vi "test_AK RS-xxx Read.vi"(8 "error in (no error)":errorcluster, 11 "TestCase in":refnum<class "Instrument Addon Serial Protocols Unit Tests.lvclass">) -> (0 "error out":errorcluster, 3 "TestCase out":refnum<class "Instrument Addon Serial Protocols Unit Tests.lvclass">)   [LabVIEW 2023, in "Instrument Addon Serial Protocols Unit Tests.lvclass"]
uses:
  Instrument Addon Serial Protocols Unit Tests.lvclass
  Instrument Addon Serial Protocols Unit Tests.lvclass/Instrument Addon Serial Protocols Unit Tests.ctl
  <vilib>/addons/_JKI Toolkits/VI Tester/TestCase.llb/TestCase.lvclass
  AK RS-xxx/AK RS-xxx.lvclass
  Protocol Parent/Methods/Read Parameter.ctl
  Protocol Parent/Protocol Parent.lvclass
  Listener/ListenerClassControls/Operation.ctl
  Listener/Listener.lvclass
  Constants.vi
  <vilib>/platform/TimedLoop/XDataNode/XDataNode.xnode
  <vilib>/Platform/TimedLoop/XDataNode/timing_clust.ctl
  <vilib>/Platform/TimedLoop/XDataNode/XDNodeRunTimeDep.lvlib
  <vilib>/Platform/TimedLoop/XDataNode/wakeup.ctl
  <vilib>/Platform/TimedLoop/XDataNode/nitl_modes.ctl
  RS-xxx/RS-xxx.lvclass
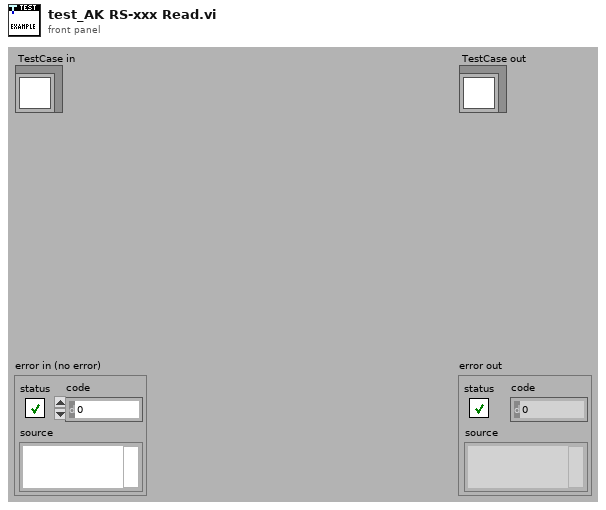
[diagram p1: front panel]
types:
  T1 = typedef "Protocols.lvlib/Protocol Parent.lvclass/Read Parameter.ctl" = cluster{"Wait Type":enum16{"Byte Count", "Wait sec"}, "Wait Value":dbl}
  T2 = typedef "Listener.lvclass/Operation.ctl" = enum16{"Read", "Write"}
  T3 = typedef "XDNodeRunTimeDep.lvlib/timing_clust.ctl" = cluster{"Expected End [f-1]":u64, "Actual End [f-1]":u64, "Finished Late? [f-1]":bool, "Expected End [i-1]":u64, "Actual End [i-1]":u64, "Finished Late? [i-1]":bool, "Expected Start [i]":u64, "Actual Start [i]":u64, "Expected Start [f]":u64, "Actual Start [f]":u64, "Source Name":string, "Structure Name":string, "Period":i64, "Deadline":i64, "Offset":i64, "Start":i64, "Priority":i32, "Timeout":i32, "Mode":T4, "Wakeup Reason":T5, "Error":errorcluster, "Source Type":string, "Secondary Source Type":string, "Global End Time":u64, "Global Start Time":u64, "Frame Duration":u64, "Iteration Duration":u64, "Assigned CPU":i32, "I/O Scan Engine Mode":u32}
  T4 = typedef "XDNodeRunTimeDep.lvlib/nitl_modes.ctl" = enum32{"No Change", "Process missed periods, maintain original phase", "Discard missed periods, maintain original phase", "Process missed periods, ignore original phase", "Discard missed periods, ignore original phase"}
  T5 = typedef "XDNodeRunTimeDep.lvlib/wakeup.ctl" = enum32{"Normal", "Aborted", "Asynchronous wakeup", "Timing source error", "Timed loop error", "Timeout"}
  T6 = typedef "Listener.lvclass/RS-xxx Data Structure.ctl" = cluster{"Virtual COM Port Settings 1":cluster{"Port":string, "Baud Rate":u32, "Data Bits":u16, "Parity":enum16{"None", "Odd", "Even", "Mark", "Space"}, "Stop Bits":u16, "Flow Control":u16, "XON":enum16{"NUL", "SOH", "STX", "ETX", "EOT", "ENQ", "ACK", "BEL", "BS", "HT", "LF", "VT", "FF", "CR", "SO", "SI", "DLE", "DC1", "DC2", "DC3", "DC4", "NAK", "SYN", "ETB", "CAN", "EM", "SUB", "ESC", "FS", "GS", "RS", "US", "SP", "!", "\"", "#", "$", "%", "&", "'", "(", ")", "*", "+", ",", "- (-)", ".", "/", "0", "1", "2", "3", "4", "5", "6", "7", "8", "9", ":", ";", "<", "=", ">", "?", "@", "A", "B", "C", "D", "E", "F", "G", "H", "I", "J", "K", "L", "M", "N", "O", "P", "Q", "R", "S", "T", "U", "V", "W", "X", "Y", "Z", "[", "\\", "]", "^", "_", "`", "a", "b", "c", "d", "e", "f", "g", "h", "i", "j", "k", "l", "m", "n", "o", "p", "q", "r", "s", "t", "u", "v", "w", "x", "y", "z", "{", "|", "}", "~"}, "XOFF":enum16{"NUL", "SOH", "STX", "ETX", "EOT", "ENQ", "ACK", "BEL", "BS", "HT", "LF", "VT", "FF", "CR", "SO", "SI", "DLE", "DC1", "DC2", "DC3", "DC4", "NAK", "SYN", "ETB", "CAN", "EM", "SUB", "ESC", "FS", "GS", "RS", "US", "SP", "!", "\"", "#", "$", "%", "&", "'", "(", ")", "*", "+", ",", "- (-)", ".", "/", "0", "1", "2", "3", "4", "5", "6", "7", "8", "9", ":", ";", "<", "=", ">", "?", "@", "A", "B", "C", "D", "E", "F", "G", "H", "I", "J", "K", "L", "M", "N", "O", "P", "Q", "R", "S", "T", "U", "V", "W", "X", "Y", "Z", "[", "\\", "]", "^", "_", "`", "a", "b", "c", "d", "e", "f", "g", "h", "i", "j", "k", "l", "m", "n", "o", "p", "q", "r", "s", "t", "u", "v", "w", "x", "y", "z", "{", "|", "}", "~"}, "End Read on Termination Character":bool, "End Write on Termination Character":bool, "Termination Character":u8}, "Virtual COM Port Settings 2":cluster{"Port":string, "Baud Rate":u32, "Data Bits":u16, "Parity":enum16{"None", "Odd", "Even", "Mark", "Space"}, "Stop Bits":u16, "Flow Control":u16, "XON":enum16{"NUL", "SOH", "STX", "ETX", "EOT", "ENQ", "ACK", "BEL", "BS", "HT", "LF", "VT", "FF", "CR", "SO", "SI", "DLE", "DC1", "DC2", "DC3", "DC4", "NAK", "SYN", "ETB", "CAN", "EM", "SUB", "ESC", "FS", "GS", "RS", "US", "SP", "!", "\"", "#", "$", "%", "&", "'", "(", ")", "*", "+", ",", "- (-)", ".", "/", "0", "1", "2", "3", "4", "5", "6", "7", "8", "9", ":", ";", "<", "=", ">", "?", "@", "A", "B", "C", "D", "E", "F", "G", "H", "I", "J", "K", "L", "M", "N", "O", "P", "Q", "R", "S", "T", "U", "V", "W", "X", "Y", "Z", "[", "\\", "]", "^", "_", "`", "a", "b", "c", "d", "e", "f", "g", "h", "i", "j", "k", "l", "m", "n", "o", "p", "q", "r", "s", "t", "u", "v", "w", "x", "y", "z", "{", "|", "}", "~"}, "XOFF":enum16{"NUL", "SOH", "STX", "ETX", "EOT", "ENQ", "ACK", "BEL", "BS", "HT", "LF", "VT", "FF", "CR", "SO", "SI", "DLE", "DC1", "DC2", "DC3", "DC4", "NAK", "SYN", "ETB", "CAN", "EM", "SUB", "ESC", "FS", "GS", "RS", "US", "SP", "!", "\"", "#", "$", "%", "&", "'", "(", ")", "*", "+", ",", "- (-)", ".", "/", "0", "1", "2", "3", "4", "5", "6", "7", "8", "9", ":", ";", "<", "=", ">", "?", "@", "A", "B", "C", "D", "E", "F", "G", "H", "I", "J", "K", "L", "M", "N", "O", "P", "Q", "R", "S", "T", "U", "V", "W", "X", "Y", "Z", "[", "\\", "]", "^", "_", "`", "a", "b", "c", "d", "e", "f", "g", "h", "i", "j", "k", "l", "m", "n", "o", "p", "q", "r", "s", "t", "u", "v", "w", "x", "y", "z", "{", "|", "}", "~"}, "End Read on Termination Character":bool, "End Write on Termination Character":bool, "Termination Character":u8}, "Data":string, "Data Length":u32}
  T7 = cluster{"Port":string, "Baud Rate":u32, "Data Bits":u16, "Parity":enum16{"None", "Odd", "Even", "Mark", "Space"}, "Stop Bits":u16, "Flow Control":u16, "XON":enum16{"NUL", "SOH", "STX", "ETX", "EOT", "ENQ", "ACK", "BEL", "BS", "HT", "LF", "VT", "FF", "CR", "SO", "SI", "DLE", "DC1", "DC2", "DC3", "DC4", "NAK", "SYN", "ETB", "CAN", "EM", "SUB", "ESC", "FS", "GS", "RS", "US", "SP", "!", "\"", "#", "$", "%", "&", "'", "(", ")", "*", "+", ",", "- (-)", ".", "/", "0", "1", "2", "3", "4", "5", "6", "7", "8", "9", ":", ";", "<", "=", ">", "?", "@", "A", "B", "C", "D", "E", "F", "G", "H", "I", "J", "K", "L", "M", "N", "O", "P", "Q", "R", "S", "T", "U", "V", "W", "X", "Y", "Z", "[", "\\", "]", "^", "_", "`", "a", "b", "c", "d", "e", "f", "g", "h", "i", "j", "k", "l", "m", "n", "o", "p", "q", "r", "s", "t", "u", "v", "w", "x", "y", "z", "{", "|", "}", "~"}, "XOFF":enum16{"NUL", "SOH", "STX", "ETX", "EOT", "ENQ", "ACK", "BEL", "BS", "HT", "LF", "VT", "FF", "CR", "SO", "SI", "DLE", "DC1", "DC2", "DC3", "DC4", "NAK", "SYN", "ETB", "CAN", "EM", "SUB", "ESC", "FS", "GS", "RS", "US", "SP", "!", "\"", "#", "$", "%", "&", "'", "(", ")", "*", "+", ",", "- (-)", ".", "/", "0", "1", "2", "3", "4", "5", "6", "7", "8", "9", ":", ";", "<", "=", ">", "?", "@", "A", "B", "C", "D", "E", "F", "G", "H", "I", "J", "K", "L", "M", "N", "O", "P", "Q", "R", "S", "T", "U", "V", "W", "X", "Y", "Z", "[", "\\", "]", "^", "_", "`", "a", "b", "c", "d", "e", "f", "g", "h", "i", "j", "k", "l", "m", "n", "o", "p", "q", "r", "s", "t", "u", "v", "w", "x", "y", "z", "{", "|", "}", "~"}, "End Read on Termination Character":bool, "End Write on Termination Character":bool, "Termination Character":u8}
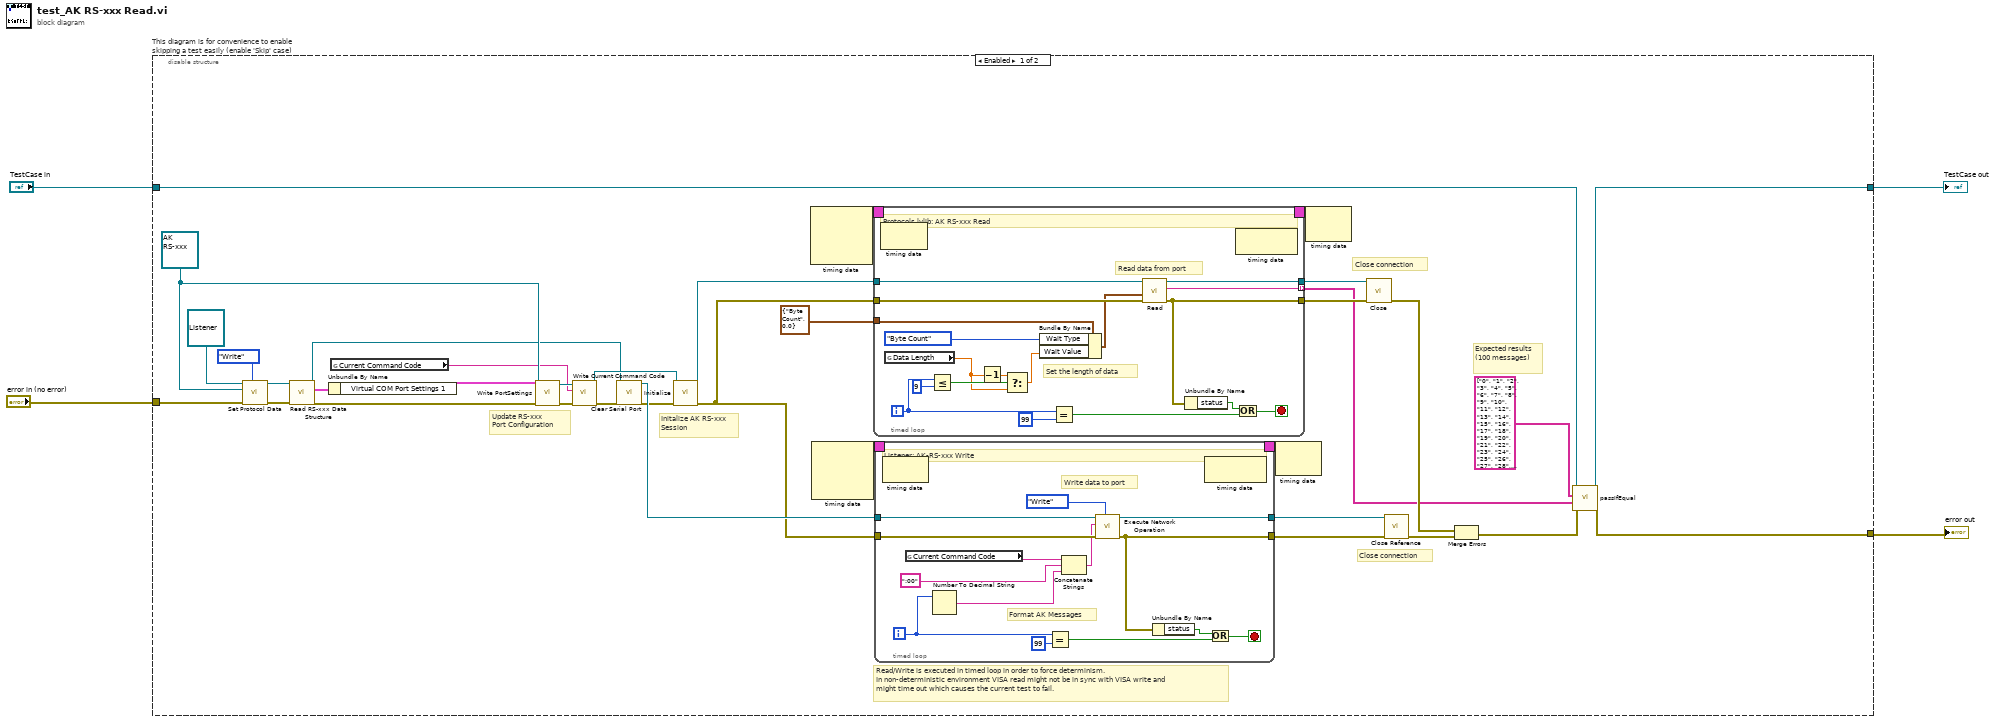
[diagram p0: block diagram]
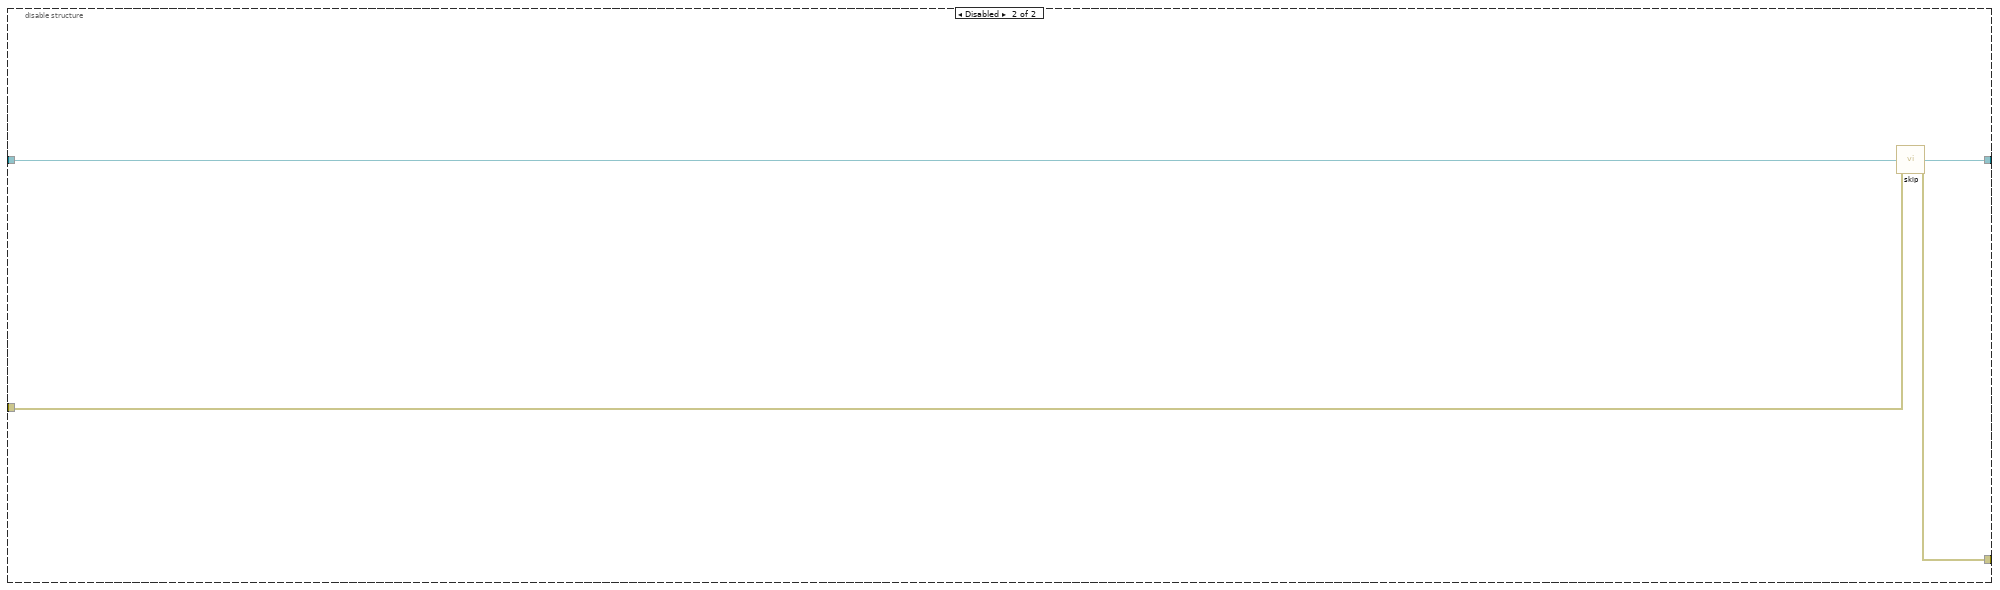
[diagram p2: hidden frame]
diagram:
  n1 = disable-structure "This diagram is for convenience to enable skipping a test easily (enable 'Skip' case)" shown="Enabled" {
    disable-tunnel: "TestCase in" -> [w40 w84]
    disable-tunnel: [w39 w82] -> w1
    disable-tunnel: [w38 w83] -> w3
    disable-tunnel: "error in (no error)" -> [w37 w81]
    frame Enabled {
      w19 = refnum<class "AK RS-xxx.lvclass"> refnum ("Protocols.lvlib:AK RS-xxx.lvclass")
      # "Update RS-xxx \nPort Configuration"
      # "Initalize AK RS-xxx\nSession"
      # "Close connection"
      # "Close connection"
      # "Expected results\n(100 messages)"
      # "Read/Write is executed in timed loop in order to force determinism.\nIn non-deterministic environment VISA read might not be in sync with VISA write and\nmight time out which causes the current test to fail."
      n2 = call "Set Protocol Data.vi"("Operation"=Operation."Write", "error in (no error)"=w37, "Protocols.lvlib:Protocol Parent.lvclass"=w19, "Listener In.lvclass"=refnum<class "Listener.lvclass"> refnum ("Listener.lvclass")) -> ("error out"=w23:errorcluster, "Listener Out.lvclass"=w24:refnum<class "Listener.lvclass">)  [unwired: 6 in]
      n3 = call-dynamic "Read RS-xxx Data Structure.vi"("error in (no error)"=w23, "Listener in"=w24) -> ("error out"=w12:errorcluster, "RS-xxx Data Structure"=w22:T6, "Listener out"=w10:refnum<class "Listener.lvclass">)  [unwired: 7 in]
      n4 = Unbundle By Name(w22) -> ("Virtual COM Port Settings 1"=w18:T7)
      n5 = global read "Constants.vi" "Current Command Code"() -> (w15:string)
      n6 = call "Write PortSettings.vi"("error in (no error)"=w12, "PortSettings"=w18, "RS232 in"=w19) -> ("error out"=w16:errorcluster, "RS232 out"=w17:refnum<class "AK RS-xxx.lvclass">)  [unwired: 7 in]
      n7 = call "Write Current Command Code.vi"("error in (no error)"=w16, "Current Command Code"=w15, "AK RS232 in"=w17) -> ("error out"=w11:errorcluster, "AK RS232 out"=w14:refnum<class "AK RS-xxx.lvclass">)  [unwired: 7 in]
      n8 = call "Clear Serial Port.vi"("error in (no error)"=w11, "Listener In.lvclass"=w10) -> ("error out"=w7:errorcluster, "Listener out"=w9:refnum<class "Listener.lvclass">)  [unwired: 8 in]
      n9 = call-dynamic "Initialize.vi"("error in (no error)"=w7, "RS232 in"=w14) -> ("error out"=w8:errorcluster, "RS232 out"=w13:refnum<class "AK RS-xxx.lvclass">)  [unwired: 8 in]
      n10 = node-c288() -> (w34:T3)  [unwired: 3 in]
      n11 = node-c288() -> (w36:T3)  [unwired: 3 in]
      n12 = timed-loop {
        timing: w34 -> [_]
        timing-out: [_] -> w33
        tunnel: T1 {"Wait Type"=enum."Byte Count", "Wait Value"=0.0} ("Read Parameter") -> [w52]
        tunnel: [w49] -> w6 mode=indexing
        tunnel: [w50] -> w20
        tunnel: w13 -> [w43]
        tunnel: w8 -> [w55]
        tunnel: [w42] -> w27
        i -> [w44]
        stop <- w56 stop-if-true
        # "Set the length of data"
        # "Read data from port"
        # "Protocols.lvlib: AK RS-xxx Read"
        n13 = node-c288() -> ()  [unwired: 1 in, 1 out]
        n14 = global read "Constants.vi" "Data Length"() -> (w48:dbl)
        n15 = Less Or Equal?(x=w44, y=9) -> (x <= y?=w53:bool)
        n16 = Decrement(x=w48) -> (x-1=w46:dbl)
        n17 = Select(t=w46, s=w53, f=w48) -> (s? t:f=w47:dbl)
        n18 = Bundle By Name(cluster=w52, "Wait Type"=enum16{"Byte Count", "Wait sec"}."Byte Count", "Wait Value"=w47) -> (w51:T1)
        n19 = Equal?(x=w44, y=99) -> (x = y?=w58:bool)
        n20 = call-dynamic "Read.vi"("error in (no error)"=w55, "Variant"=w51, "AK RS232 in"=w43) -> ("error out"=w42:errorcluster, "String"=w49:string, "AK RS232 out"=w50:refnum<class "AK RS-xxx.lvclass">)  [unwired: 6 in]
        n21 = Unbundle By Name(w42) -> ("status"=w41:bool)
        n22 = node-c288() -> ()  [unwired: 1 in, 1 out]
        n23 = Or(x=w41, y=w58) -> (x .or. y?=w56:bool)
      }
      n24 = timed-loop {
        timing: w36 -> [_]
        timing-out: [_] -> w35
        tunnel: w9 -> [w72]
        tunnel: [w73] -> w26
        tunnel: w8 -> [w71]
        tunnel: [w64] -> w25
        i -> [w67]
        stop <- w74 stop-if-true
        # "Format AK Messages"
        # "Write data to port"
        # "Listener: AK-RS-xxx Write"
        n25 = node-c288() -> ()  [unwired: 1 in, 1 out]
        n26 = global read "Constants.vi" "Current Command Code"() -> (w68:string)
        n27 = Number To Decimal String(number=w67) -> (decimal integer string=w69:string)  [unwired: 1 in]
        n28 = Equal?(x=w67, y=99) -> (x = y?=w75:bool)
        n29 = Concatenate Strings(w68, ":00", w69) -> (w66:string)
        n30 = call "Execute Network Operation.vi"("Operation"=Operation."Write", "error in (no error)"=w71, "Message"=w66, "Listener In.lvclass"=w72) -> ("error out"=w64:errorcluster, "Listener Out.lvclass"=w73:refnum<class "Listener.lvclass">)  [unwired: 6 in]
        n31 = Unbundle By Name(w64) -> ("status"=w63:bool)
        n32 = node-c288() -> ()  [unwired: 1 in, 1 out]
        n33 = Or(x=w63, y=w75) -> (x .or. y?=w74:bool)
      }
      n34 = node-c288(w35) -> ()  [unwired: 1 out]
      n35 = node-c288(w33) -> ()  [unwired: 1 out]
      n36 = call-dynamic "Close.vi"("error in (no error)"=w27, "RS232 in"=w20) -> ("error out"=w29:errorcluster)  [unwired: 8 in, 1 out]
      n37 = call "Close Reference.vi"("error in (no error)"=w25, "Listener In.lvclass"=w26) -> ("error out"=w28:errorcluster)  [unwired: 8 in, 1 out]
      n38 = Merge Errors(w29, w28) -> (w30:errorcluster)
      n39 = call-dynamic "passIfEqual.vi"("error in (no error)"=w30, "y"=w6, "x"=string[] ["0", "1", "2", "3", "4", "5", "6", "7", "8", "9", "10", "11", "12", "13", "14", "15", "16", "17", "18", "19", "20", "21", "22", "23", "24", "25", "26", "27", "28", "29", "30", "31", "32", "33", "34", "35", "36", "37", "38", "39", "40", "41", "42", "43", "44", "45", "46", "47", "48", "49", "50", "51", "52", "53", "54", "55", "56", "57", "58", "59", "60", "61", "62", "63", "64", "65", "66", "67", "68", "69", "70", "71", "72", "73", "74", "75", "76", "77", "78", "79", "80", "81", "82", "83", "84", "85", "86", "87", "88", "89", "90", "91", "92", "93", "94", "95", "96", "97", "98", "99"] ("Array"), "TestCase in"=w40) -> ("error out"=w38:errorcluster, "TestCase out"=w39:refnum<class "Instrument Addon Serial Protocols Unit Tests.lvclass">)  [unwired: 6 in]
    }
    frame Disabled {
      # "skip test result while test is under development"
      n40 = call <vilib>:"skip.vi"("error in (no error)"=w81, "TestCase in"=w84) -> ("error out"=w83:errorcluster, "TestCase out"=w82:refnum<class "Instrument Addon Serial Protocols Unit Tests.lvclass">)  [unwired: 8 in]
    }
  }
  "error out" <- w3
  "TestCase out" <- w1
